vi "Init.vi"(8 "Error In":errorcluster, 11 "ComboBox Ref":refnum<vi>) -> (0 "Error Out":errorcluster)   [LabVIEW 2023, in "Error Manager.lvlib" / "Display Order Combo Box.lvclass"]
doc: "Blank VI with error handling."
uses:
  Private VIs/Display Order (enum).ctl
  Display Order Combo Box.lvclass
  Display Order Combo Box.lvclass/Display Order Combo Box.ctl
  Error Manager.lvlib
panel:
  out "ComboBox Strings":string[](array[string])
  # "Input\nInputs to the VI"
  # "Development\nControls or indicators that are useful for development or testing, but which are not outputs of the VI."
  # "Output\nOutputs of the VI"
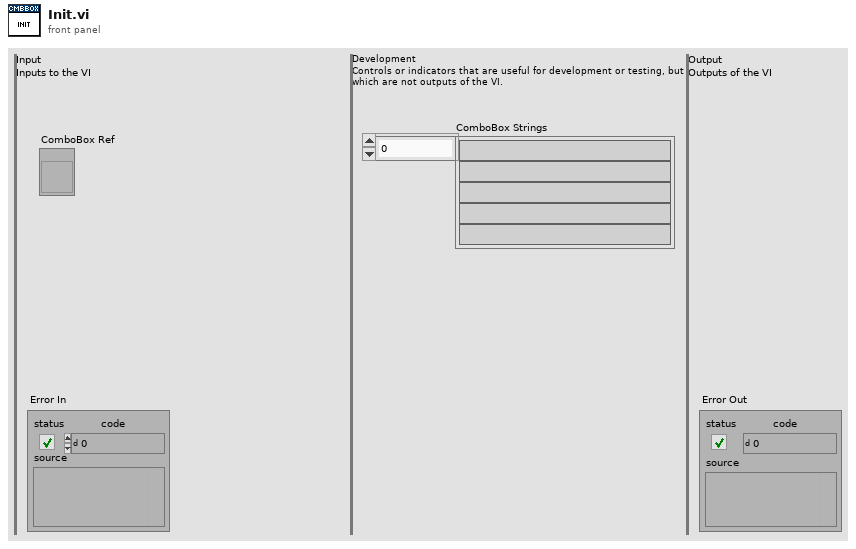
[diagram p1: front panel]
types:
  T1 = typedef "Error Manager.lvlib/Display Order (enum).ctl" = enum16{"Most Recent First (inverse-chronological)", "Oldest First (chronological)"}
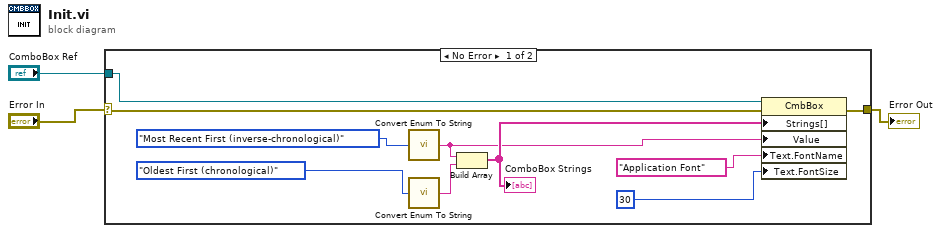
[diagram p0: block diagram]
diagram:
  n1 = case shown="No Error" "Error In" {
    selector: "Error In" -> [w13 w14]
    tunnel: [w7 w14] -> w2
    tunnel: "ComboBox Ref" -> [w12 _]
    frame No Error {
      n2 = call "Convert Enum To String.vi"("Display Order (enum)"=Display_Order_(enum)."Most Recent First (inverse-chronological)" ("Display Order")) -> ("Display Order (ComboBox string)"=w6:string)
      n3 = call "Convert Enum To String.vi"("Display Order (enum)"=Display_Order_(enum)."Oldest First (chronological)" ("Display Order")) -> ("Display Order (ComboBox string)"=w9:string)
      n4 = Build Array(w6, w9) -> (w8:string[])
      "ComboBox Strings" <- w8
      n5 = property class="CmbBox"(reference=w12, error in=w13, "Strings[]"=w8, "Value"=w6, "Text.FontName"="Application Font" ("Text.Font:Name"), "Text.FontSize"=u32 30 ("Text.Font:Size")) -> (error out=w7:errorcluster)  [unwired: 1 out]
    }
    frame Error {
    }
  }
  "Error Out" <- w2
